vi "CSDB_Config.main.vi"(5 "error in (no error)":errorcluster) -> ()   [LabVIEW 2014, in "CSDB_Config.lvlib"]
doc: "Main User Panel"
uses:
  CSDB_Config.lvlib
panel:
  in  "select all":bool
  in  "delete instances":bool
  in  "cFilter :":string caption="Filter :"
  in  "createCSVFile4SVs":bool
  in  "Filter :":string
  out "Selected Instance :":string
  in  "edit selected instances":bool
  out "error out":errorcluster
  in  "exit":bool
  in  "createWithDefault":bool
  in  "create":bool
  in  "Preview":i32(listbox)
  in  "Instances":i32[](listbox)
  in  "Classes":i32(listbox)
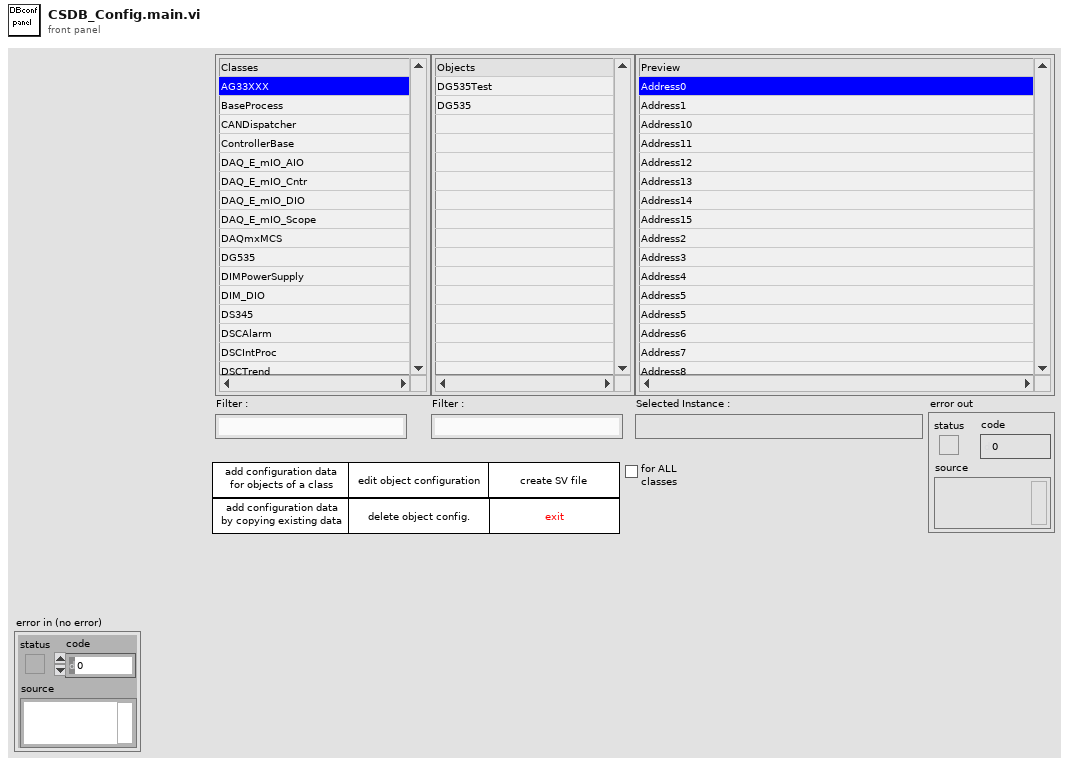
[diagram p1: front panel]
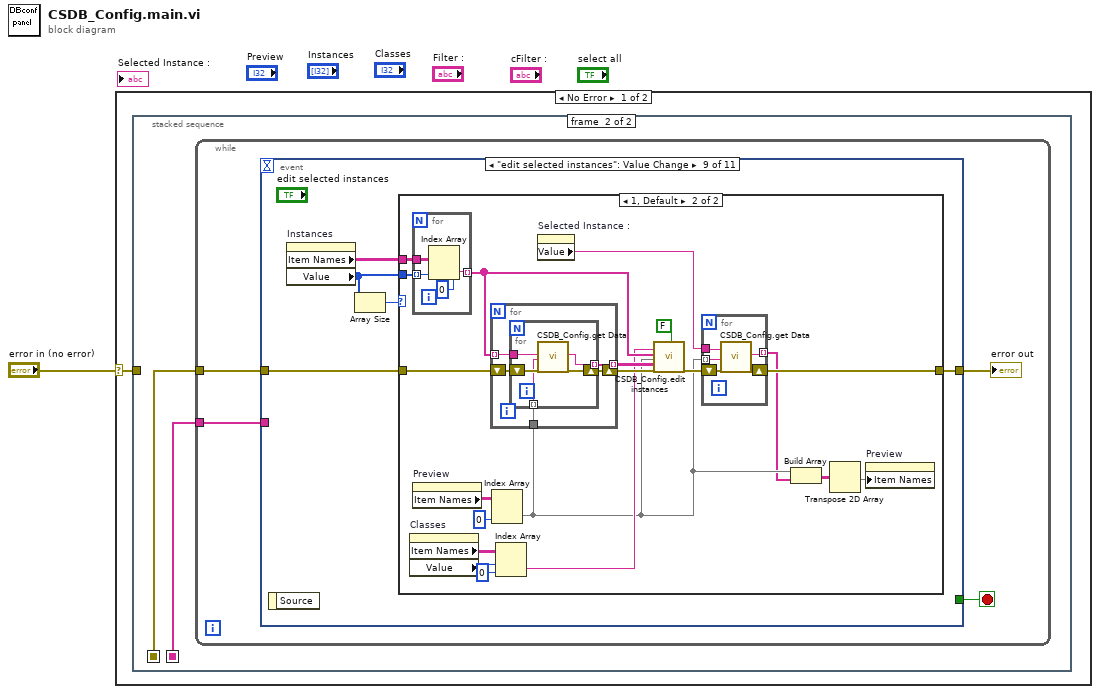
[diagram p0: block diagram]
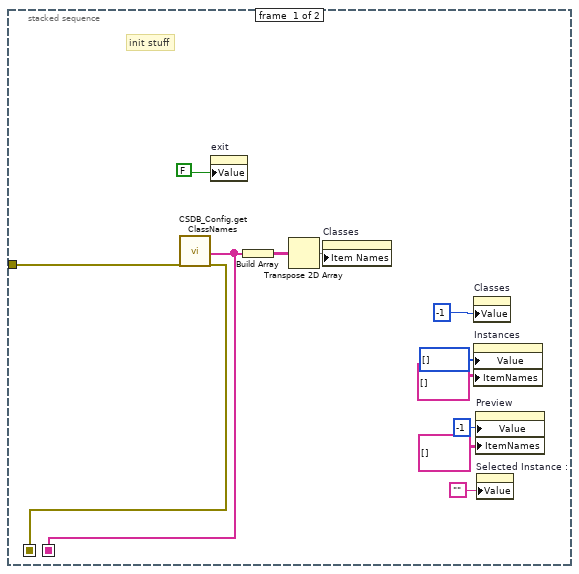
[diagram p2: hidden frame]
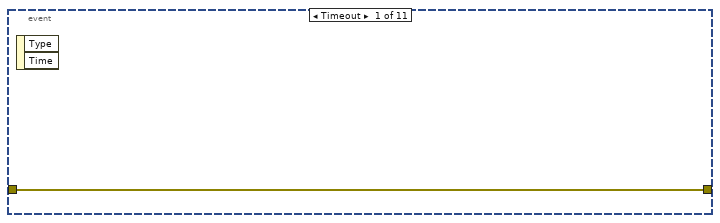
[diagram p3: hidden frame]
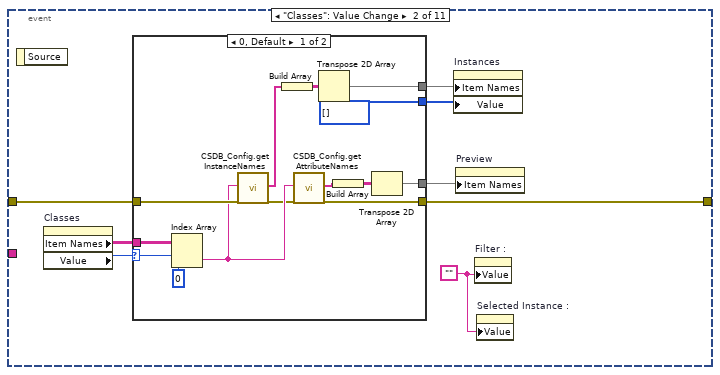
[diagram p4: hidden frame]
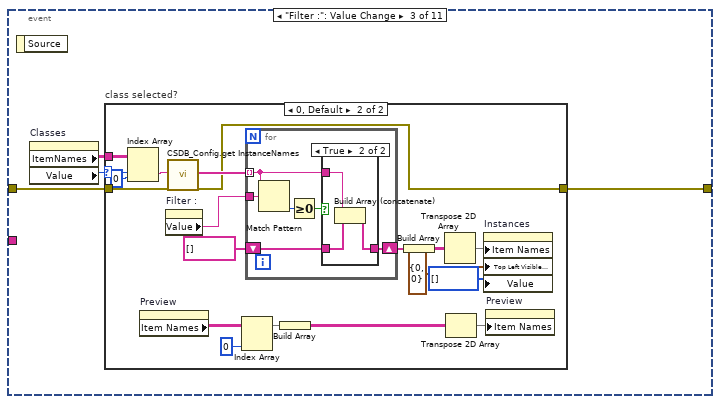
[diagram p6: hidden frame]
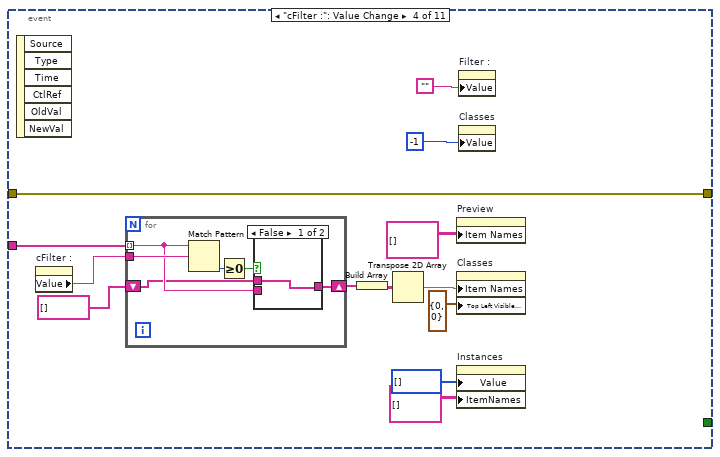
[diagram p9: hidden frame]
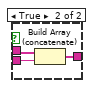
[diagram p10: hidden frame]
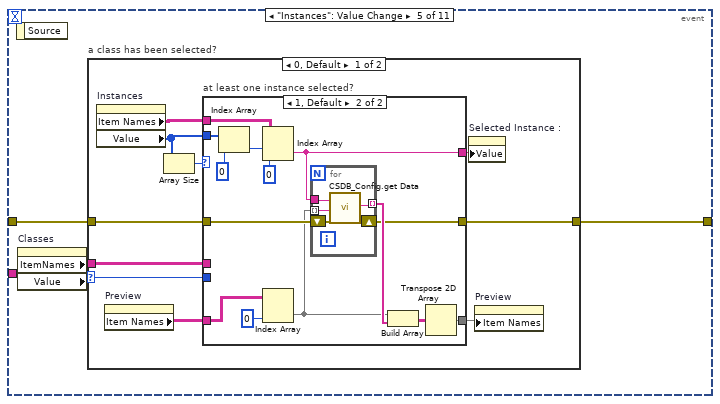
[diagram p11: hidden frame]
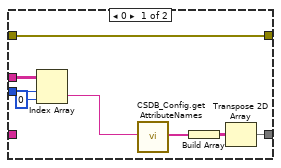
[diagram p12: hidden frame]
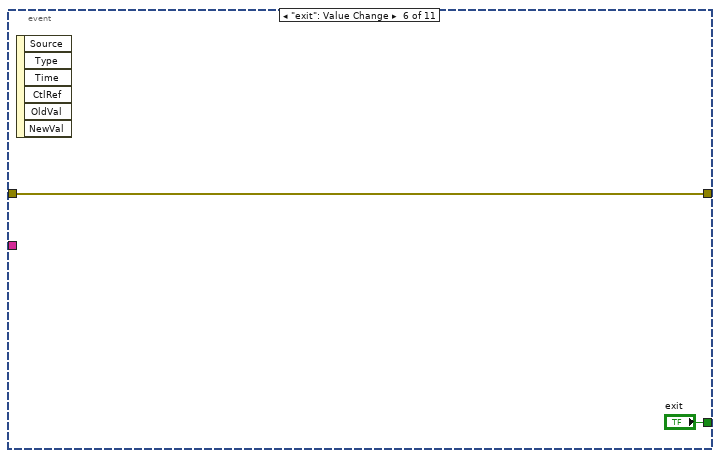
[diagram p14: hidden frame]
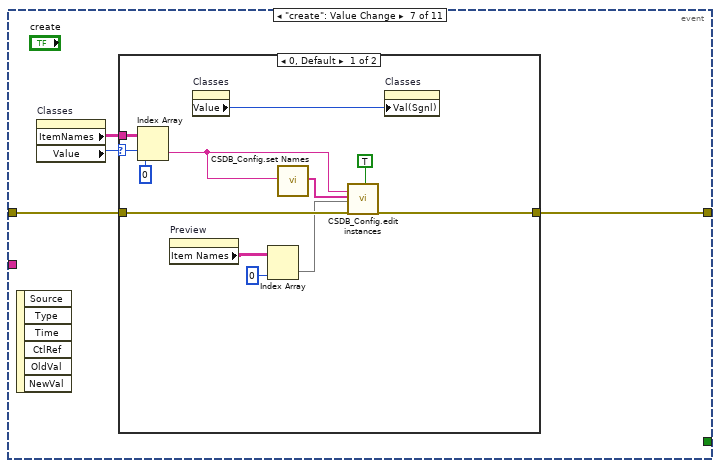
[diagram p15: hidden frame]
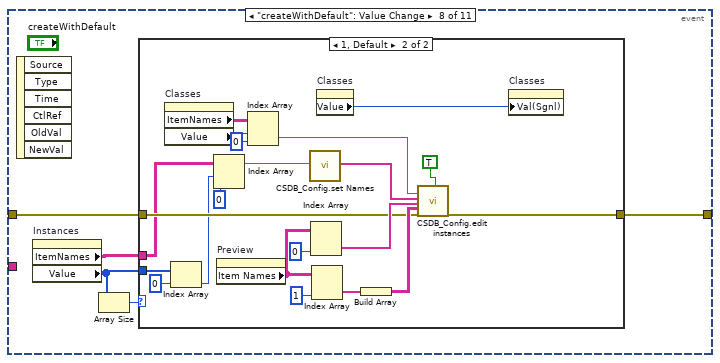
[diagram p17: hidden frame]
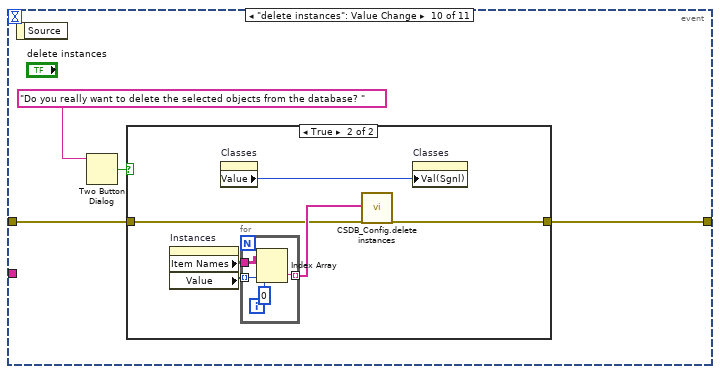
[diagram p20: hidden frame]
diagram:
  n1 = case shown="No Error" "error in (no error)" {
    selector: "error in (no error)" -> [w2 w288]
    frame No Error {
      n2 = stacked-sequence {
        seq-local: [w12 _] -> [_ w16]
        seq-local: [w7 _] -> [_ w15]
        tunnel: w2 -> [w13 _]
        frame #0 {
          # "init stuff"
          n3 = call "CSDB_Config.get ClassNames.vi"("error in (no error)"=w13) -> ("ClassNames"=w7:string[], "error out"=w12:errorcluster)  [unwired: 17 in]
          n4 = property on="exit" class="Bool"("Value"=FALSE) -> ()  [unwired: 2 in, 2 out]
          n5 = Build Array(w7) -> (w6:string[][])
          n6 = Transpose 2D Array(2D array=w6) -> (transposed array=w14:string[][])
          n7 = property on="Classes" class="MCListbox (strict)"("Item Names"=w14) -> ()  [unwired: 2 in, 2 out]
          n8 = property on="Classes" class="MCListbox (strict)"("Value"=-1 ("Classes")) -> ()  [unwired: 2 in, 2 out]
          n9 = property on="Instances" class="MCListbox (strict)"("Value"=i32[] [] ("Instances"), "ItemNames"=string[][] [] ("Item Names")) -> ()  [unwired: 2 in, 2 out]
          n10 = property on="Preview" class="MCListbox (strict)"("Value"=-1 ("Preview"), "ItemNames"=string[][] [] ("Item Names")) -> ()  [unwired: 2 in, 2 out]
          n11 = property on="Selected Instance :" class="Str"("Value"="") -> ()  [unwired: 2 in, 2 out]
        }
        frame #1 {
          n12 = while {
            tunnel: w16 -> [w19]
            tunnel: w15 -> [w18]
            stop <- w20 stop-if-true
            n13 = event shown="[8] \"edit selected instances\": Value Change" {
              selector: _ -> [_ _ _ _ _ _ _ _ _ _ _]
              dyn-events: _ -> [_ _ _ _ _ _ _ _ _ _ _]
              timeout: _ -> [_ _ _ _ _ _ _ _ _ _ _]
              tunnel: [_ _ _ _ _ "exit" _ _ _ _ _] -> w20
              tunnel: w19 -> [w21 w28 w48 w79 w105 w144 w149 w167 w193 w238 w253]
              tunnel: w18 -> [_ _ _ w91 _ _ _ _ _ _ w255]
              tunnel: [w21 w27 w45 w79 w103 w144 w146 w163 w190 w235 w251] -> w17
              event Timeout {
                n14 = event-data() -> ()  [unwired: 1 in, 2 out]
              }
              event "Classes": Value Change {
                w23 = ""
                n15 = event-data() -> ()  [unwired: 1 in, 1 out]
                n16 = property on="Classes" class="MCListbox (strict)"() -> ("Item Names"=w29:string[][], "Value"=w22:i32)  [unwired: 2 in, 2 out]
                n17 = case shown="0, Default" w22 {
                  selector: w22 -> [w30 _]
                  tunnel: w29 -> [w43 _]
                  tunnel: w28 -> [w42 w44]
                  tunnel: [w41 w44] -> w27
                  tunnel: [w37 _] -> w26
                  tunnel: [i32[] [] ("Instances") _] -> w25
                  tunnel: [w32 _] -> w24
                  frame 0, Default {
                    n18 = Index Array(array=w43, index (row)=w30, index (col)=0 ("disabled index (col)")) -> (element=w35:string)
                    n19 = call "CSDB_Config.get InstanceNames.vi"("ClassName"=w35, "error in (no error)"=w42) -> ("InstanceNames"=w39:string[], "error out"=w31:errorcluster)  [unwired: 16 in]
                    n20 = Build Array(w39) -> (w38:string[][])
                    n21 = call "CSDB_Config.get AttributeNames.vi"("ClassName"=w35, "error in (no error)"=w31) -> ("Attribute"=w34:string[], "error out"=w41:errorcluster)  [unwired: 16 in]
                    n22 = Transpose 2D Array(2D array=w38) -> (transposed array=w37:string[][])
                    n23 = Build Array(w34) -> (w33:string[][])
                    n24 = Transpose 2D Array(2D array=w33) -> (transposed array=w32:string[][])
                  }
                  frame -1 {
                  }
                }
                n25 = property on="Instances" class="MCListbox (strict)"("Item Names"=w26, "Value"=w25) -> ()  [unwired: 2 in, 2 out]
                n26 = property on="Preview" class="MCListbox (strict)"("Item Names"=w24) -> ()  [unwired: 2 in, 2 out]
                n27 = property on="Filter :" class="Str"("Value"=w23) -> ()  [unwired: 2 in, 2 out]
                n28 = property on="Selected Instance :" class="Str"("Value"=w23) -> ()  [unwired: 2 in, 2 out]
              }
              event "Filter :": Value Change {
                n29 = event-data() -> ()  [unwired: 1 in, 1 out]
                n30 = property on="Classes" class="MCListbox (strict)"() -> ("ItemNames"=w46:string[][], "Value"=w47:i32)  [unwired: 2 in, 2 out]
                n31 = case "class selected?" shown="0, Default" w47 {
                  selector: w47 -> [_ w59]
                  tunnel: w48 -> [w49 w68]
                  tunnel: w46 -> [_ w60]
                  tunnel: [w49 w50] -> w45
                  frame -1 {
                  }
                  frame 0, Default {
                    n32 = Index Array(array=w60, index (row)=w59, index (col)=0 ("disabled index (col)")) -> (element=w57:string)
                    n33 = property on="Preview" class="MCListbox (strict)"() -> ("Item Names"=w55:string[][])  [unwired: 2 in, 2 out]
                    n34 = property on="Filter :" class="Str"() -> ("Value"=w56:string)  [unwired: 2 in, 2 out]
                    n35 = call "CSDB_Config.get InstanceNames.vi"("ClassName"=w57, "error in (no error)"=w68) -> ("InstanceNames"=w67:string[], "error out"=w50:errorcluster)  [unwired: 16 in]
                    n36 = Index Array(array=w55, index (col)=0 ("disabled index (col)")) -> (element=w53:string[])  [unwired: 1 in]
                    n37 = for {
                      tunnel: w67 -> [w71] mode=indexing
                      tunnel: w56 -> [w74]
                      shift-right: [w69] -> w64
                      shift-left: string[] [] -> [w70]
                      n38 = Match Pattern(string=w71, regular expression=w74) -> (offset past match=w73:i32)  [unwired: 1 in, 3 out]
                      n39 = Greater Or Equal To 0?(x=w73) -> (x >= 0?=w72:bool)
                      n40 = case shown="True" w72 {
                        tunnel: w71 -> [_ w78]
                        tunnel: w70 -> [w75 w77]
                        tunnel: [w75 w76] -> w69
                        frame False {
                        }
                        frame True {
                          n41 = Build Array (concatenate)(w77, w78) -> (w76:string[])
                        }
                      }
                    }
                    n42 = Build Array(w53) -> (w52:string[][])
                    n43 = Build Array(w64) -> (w65:string[][])
                    n44 = Transpose 2D Array(2D array=w65) -> (transposed array=w63:string[][])
                    n45 = Transpose 2D Array(2D array=w52) -> (transposed array=w51:string[][])
                    n46 = property on="Instances" class="MCListbox (strict)"("Item Names"=w63, "Top Left Visible Cell"=cluster{"Row":u32, "Column":u32} {"Row"=0, "Column"=0}, "Value"=i32[] [] ("Instances")) -> ()  [unwired: 2 in, 2 out]
                    n47 = property on="Preview" class="MCListbox (strict)"("Item Names"=w51) -> ()  [unwired: 2 in, 2 out]
                  }
                }
              }
              event "cFilter :": Value Change {
                n48 = event-data() -> ()  [unwired: 1 in, 6 out]
                n49 = property on="cFilter :" class="Str"() -> ("Value"=w80:string)  [unwired: 2 in, 2 out]
                n50 = for {
                  tunnel: w91 -> [w94] mode=indexing
                  tunnel: w80 -> [w97]
                  shift-right: [w93] -> w88
                  shift-left: string[] [] -> [w92]
                  n51 = Match Pattern(string=w94, regular expression=w97) -> (offset past match=w96:i32)  [unwired: 1 in, 3 out]
                  n52 = Greater Or Equal To 0?(x=w96) -> (x >= 0?=w95:bool)
                  n53 = case shown="False" w95 {
                    tunnel: w94 -> [_ w101]
                    tunnel: [w98 w100] -> w93
                    tunnel: w92 -> [w98 w99]
                    frame False {
                    }
                    frame True {
                      n54 = Build Array (concatenate)(w99, w101) -> (w100:string[])
                    }
                  }
                }
                n55 = Build Array(w88) -> (w89:string[][])
                n56 = Transpose 2D Array(2D array=w89) -> (transposed array=w87:string[][])
                n57 = property on="Preview" class="MCListbox (strict)"("Item Names"=string[][] []) -> ()  [unwired: 2 in, 2 out]
                n58 = property on="Classes" class="MCListbox (strict)"("Item Names"=w87, "Top Left Visible Cell"=cluster{"Row":u32, "Column":u32} {"Row"=0, "Column"=0}) -> ()  [unwired: 2 in, 2 out]
                n59 = property on="Instances" class="MCListbox (strict)"("Value"=i32[] [] ("Instances"), "ItemNames"=string[][] [] ("Item Names")) -> ()  [unwired: 2 in, 2 out]
                n60 = property on="Filter :" class="Str"("Value"="") -> ()  [unwired: 2 in, 2 out]
                n61 = property on="Classes" class="MCListbox (strict)"("Value"=-1 ("Classes")) -> ()  [unwired: 2 in, 2 out]
              }
              event "Instances": Value Change {
                n62 = event-data() -> ()  [unwired: 1 in, 1 out]
                n63 = property on="Classes" class="MCListbox (strict)"() -> ("ItemNames"=w102:string[][], "Value"=w104:i32)  [unwired: 2 in, 2 out]
                n64 = case "a class has been selected?" shown="0, Default" w104 {
                  selector: w104 -> [w106 _]
                  tunnel: w105 -> [w114 w143]
                  tunnel: [w111 w143] -> w103
                  tunnel: w102 -> [w107 _]
                  frame 0, Default {
                    n65 = property on="Instances" class="MCListbox (strict)"() -> ("Item Names"=w115:string[][], "Value"=w109:i32[])  [unwired: 2 in, 2 out]
                    n66 = property on="Preview" class="MCListbox (strict)"() -> ("Item Names"=w108:string[][])  [unwired: 2 in, 2 out]
                    n67 = Array Size(array=w109) -> (size(s)=w110:i32)
                    n68 = case "at least one instance selected?" shown="1, Default" w110 {
                      tunnel: w115 -> [_ w137]
                      tunnel: w114 -> [w123 w135]
                      tunnel: [w120 w132] -> w113
                      tunnel: [_ w129] -> w112
                      tunnel: w109 -> [_ w128]
                      tunnel: [w123 w125] -> w111
                      tunnel: w108 -> [_ w124]
                      tunnel: w107 -> [w119 _]
                      tunnel: w106 -> [w118 _]
                      frame 0 {
                        n69 = Index Array(array=w119, index (row)=w118, index (col)=0 ("disabled index (col)")) -> (element=w116:string)
                        n70 = call "CSDB_Config.get AttributeNames.vi"("ClassName"=w116) -> ("Attribute"=w122:string[])  [unwired: 17 in, 1 out]
                        n71 = Build Array(w122) -> (w121:string[][])
                        n72 = Transpose 2D Array(2D array=w121) -> (transposed array=w120:string[][])
                      }
                      frame 1, Default {
                        n73 = Index Array(array=w128, index=0) -> (element=w131:i32)
                        n74 = Index Array(array=w137, index (row)=w131, index (col)=0 ("disabled index (col)")) -> (element=w129:string)
                        n75 = Index Array(array=w124, index (col)=0 ("disabled index (col)")) -> (element=w126:string[])  [unwired: 1 in]
                        n76 = for {
                          tunnel: w129 -> [w141]
                          tunnel: w126 -> [w140] mode=indexing
                          tunnel: [w139] -> w134 mode=indexing
                          shift-right: [w138] -> w125
                          shift-left: w135 -> [w142]
                          n77 = call "CSDB_Config.get Data.vi"("InstanceName"=w141, "AttributeName"=w140, "error in (no error)"=w142) -> ("Value"=w139:string, "error out"=w138:errorcluster)  [unwired: 15 in]
                        }
                        n78 = Build Array(w126, w134) -> (w133:string[][])
                        n79 = Transpose 2D Array(2D array=w133) -> (transposed array=w132:string[][])
                      }
                    }
                    n80 = property on="Selected Instance :" class="Str"("Value"=w112) -> ()  [unwired: 2 in, 2 out]
                    n81 = property on="Preview" class="MCListbox (strict)"("Item Names"=w113) -> ()  [unwired: 2 in, 2 out]
                  }
                  frame -1 {
                  }
                }
              }
              event "exit": Value Change {
                n82 = event-data() -> ()  [unwired: 1 in, 6 out]
              }
              event "create": Value Change {
                n83 = event-data() -> ()  [unwired: 1 in, 6 out]
                n84 = property on="Classes" class="MCListbox (strict)"() -> ("ItemNames"=w147:string[][], "Value"=w148:i32)  [unwired: 2 in, 2 out]
                n85 = case shown="0, Default" w148 {
                  selector: w148 -> [w157 _]
                  tunnel: w149 -> [w159 w162]
                  tunnel: w147 -> [w158 _]
                  tunnel: [w151 w162] -> w146
                  frame 0, Default {
                    n86 = Index Array(array=w158, index (row)=w157, index (col)=0 ("disabled index (col)")) -> (element=w155:string)
                    n87 = property on="Preview" class="MCListbox (strict)"() -> ("Item Names"=w154:string[][])  [unwired: 2 in, 2 out]
                    n88 = property on="Classes" class="MCListbox (strict)"() -> ("Value"=w150:i32)  [unwired: 2 in, 2 out]
                    n89 = Index Array(array=w154, index (col)=0 ("disabled index (col)")) -> (element=w152:string[])  [unwired: 1 in]
                    n90 = call "CSDB_Config.set Names.vi"("Name"=w155) -> ("Names"=w161:string[])  [unwired: 18 in]
                    n91 = call "CSDB_Config.edit instances.vi"("Classname"=w155, "Names"=w161, "Attributes"=w152, "error in (no error)"=w159, "new instances?"=TRUE) -> ("error out"=w151:errorcluster)  [unwired: 14 in]
                    n92 = property on="Classes" class="MCListbox (strict)"("Val(Sgnl)"=w150) -> ()  [unwired: 2 in, 2 out]
                  }
                  frame -1 {
                  }
                }
              }
              event "createWithDefault": Value Change {
                n93 = event-data() -> ()  [unwired: 1 in, 6 out]
                n94 = property on="Instances" class="MCListbox (strict)"() -> ("ItemNames"=w164:string[][], "Value"=w165:i32[])  [unwired: 2 in, 2 out]
                n95 = Array Size(array=w165) -> (size(s)=w166:i32)
                n96 = case shown="1, Default" w166 {
                  tunnel: w167 -> [w168 w181]
                  tunnel: w165 -> [_ w178]
                  tunnel: w164 -> [_ w177]
                  tunnel: [w168 w170] -> w163
                  frame 0 {
                  }
                  frame 1, Default {
                    n97 = property on="Classes" class="MCListbox (strict)"() -> ("ItemNames"=w174:string[][], "Value"=w173:i32)  [unwired: 2 in, 2 out]
                    n98 = Index Array(array=w178, index=0) -> (element=w179:i32)
                    n99 = Index Array(array=w177, index (row)=w179, index (col)=0 ("disabled index (col)")) -> (element=w176:string)
                    n100 = property on="Preview" class="MCListbox (strict)"() -> ("Item Names"=w185:string[][])  [unwired: 2 in, 2 out]
                    n101 = Index Array(array=w174, index (row)=w173, index (col)=0 ("disabled index (col)")) -> (element=w171:string)
                    n102 = call "CSDB_Config.set Names.vi"("Name"=w176) -> ("Names"=w189:string[])  [unwired: 18 in]
                    n103 = Index Array(array=w185, index (col)=0 ("disabled index (col)")) -> (element=w188:string[])  [unwired: 1 in]
                    n104 = Index Array(array=w185, index (col)=1 ("disabled index (col)")) -> (element=w184:string[])  [unwired: 1 in]
                    n105 = property on="Classes" class="MCListbox (strict)"() -> ("Value"=w169:i32)  [unwired: 2 in, 2 out]
                    n106 = Build Array(w184) -> (w183:string[][])
                    n107 = call "CSDB_Config.edit instances.vi"("Classname"=w171, "Names"=w189, "Attributes"=w188, "Values"=w183, "error in (no error)"=w181, "new instances?"=TRUE) -> ("error out"=w170:errorcluster)  [unwired: 13 in]
                    n108 = property on="Classes" class="MCListbox (strict)"("Val(Sgnl)"=w169) -> ()  [unwired: 2 in, 2 out]
                  }
                }
              }
              event "edit selected instances": Value Change {
                n109 = event-data() -> ()  [unwired: 1 in, 1 out]
                n110 = property on="Instances" class="MCListbox (strict)"() -> ("Item Names"=w194:string[][], "Value"=w192:i32[])  [unwired: 2 in, 2 out]
                n111 = Array Size(array=w192) -> (size(s)=w191:i32)
                n112 = case shown="1, Default" w191 {
                  tunnel: w192 -> [_ w215]
                  tunnel: w194 -> [_ w214]
                  tunnel: w193 -> [w195 w207]
                  tunnel: [w195 w201] -> w190
                  frame 0 {
                  }
                  frame 1, Default {
                    n113 = property on="Classes" class="MCListbox (strict)"() -> ("Item Names"=w206:string[][], "Value"=w205:i32)  [unwired: 2 in, 2 out]
                    n114 = for {
                      tunnel: w215 -> [w233] mode=indexing
                      tunnel: w214 -> [w234]
                      tunnel: [w231] -> w210 mode=indexing
                      n115 = Index Array(array=w234, index (row)=w233, index (col)=0 ("disabled index (col)")) -> (element=w231:string)
                    }
                    n116 = property on="Preview" class="MCListbox (strict)"() -> ("Item Names"=w213:string[][])  [unwired: 2 in, 2 out]
                    n117 = Index Array(array=w213, index (col)=0 ("disabled index (col)")) -> (element=w198:string[])  [unwired: 1 in]
                    n118 = for {
                      tunnel: w210 -> [w223] mode=indexing
                      tunnel: w198 -> [w222]
                      tunnel: [w221] -> w209 mode=indexing
                      shift-right: [w224] -> w211
                      shift-left: w207 -> [w225]
                      n119 = for {
                        tunnel: w223 -> [w228]
                        tunnel: w222 -> [w227] mode=indexing
                        tunnel: [w226] -> w221 mode=indexing
                        shift-right: [w229] -> w224
                        shift-left: w225 -> [w230]
                        n120 = call "CSDB_Config.get Data.vi"("InstanceName"=w228, "AttributeName"=w227, "error in (no error)"=w230) -> ("Value"=w226:string, "error out"=w229:errorcluster)  [unwired: 15 in]
                      }
                    }
                    n121 = Index Array(array=w206, index (row)=w205, index (col)=0 ("disabled index (col)")) -> (element=w203:string)
                    n122 = property on="Selected Instance :" class="Str"() -> ("Value"=w200:string)  [unwired: 2 in, 2 out]
                    n123 = call "CSDB_Config.edit instances.vi"("Classname"=w203, "Names"=w210, "Attributes"=w198, "Values"=w209, "error in (no error)"=w211, "new instances?"=FALSE) -> ("error out"=w202:errorcluster)  [unwired: 13 in]
                    n124 = for {
                      tunnel: w200 -> [w219]
                      tunnel: w198 -> [w218] mode=indexing
                      tunnel: [w217] -> w197 mode=indexing
                      shift-right: [w216] -> w201
                      shift-left: w202 -> [w220]
                      n125 = call "CSDB_Config.get Data.vi"("InstanceName"=w219, "AttributeName"=w218, "error in (no error)"=w220) -> ("Value"=w217:string, "error out"=w216:errorcluster)  [unwired: 15 in]
                    }
                    n126 = Build Array(w198, w197) -> (w199:string[][])
                    n127 = Transpose 2D Array(2D array=w199) -> (transposed array=w196:string[][])
                    n128 = property on="Preview" class="MCListbox (strict)"("Item Names"=w196) -> ()  [unwired: 2 in, 2 out]
                  }
                }
              }
              event "delete instances": Value Change {
                n129 = event-data() -> ()  [unwired: 1 in, 1 out]
                n130 = Two Button Dialog(message="Do you really want to delete the selected objects from the database? ") -> (T button?=w237:bool)  [unwired: 2 in]
                n131 = case shown="True" w237 {
                  tunnel: w238 -> [w239 w242]
                  tunnel: [w239 w241] -> w235
                  frame False {
                  }
                  frame True {
                    n132 = property on="Instances" class="MCListbox (strict)"() -> ("Item Names"=w244:string[][], "Value"=w245:i32[])  [unwired: 2 in, 2 out]
                    n133 = property on="Classes" class="MCListbox (strict)"() -> ("Value"=w240:i32)  [unwired: 2 in, 2 out]
                    n134 = for {
                      tunnel: w245 -> [w248] mode=indexing
                      tunnel: w244 -> [w249]
                      tunnel: [w246] -> w243 mode=indexing
                      n135 = Index Array(array=w249, index (row)=w248, index (col)=0 ("disabled index (col)")) -> (element=w246:string)
                    }
                    n136 = call "CSDB_Config.delete instances.vi"("Names"=w243, "error in (no error)"=w242) -> ("error out"=w241:errorcluster)  [unwired: 17 in]
                    n137 = property on="Classes" class="MCListbox (strict)"("Val(Sgnl)"=w240) -> ()  [unwired: 2 in, 2 out]
                  }
                }
              }
              event "createCSVFile4SVs": Value Change {
                n138 = event-data() -> ()  [unwired: 1 in, 6 out]
                n139 = property on="select all" class="Bool (strict)"() -> ("Value"=w250:bool)  [unwired: 2 in, 2 out]
                n140 = case "for ALL objects?" shown="False" w250 {
                  tunnel: [w262 w276] -> w256
                  tunnel: w255 -> [_ w277]
                  tunnel: cluster{string, string}[] [] -> [_ w275]
                  tunnel: w253 -> [w257 w274]
                  tunnel: [w257 w273] -> w252
                  frame False {
                    n141 = property on="Instances" class="MCListbox (strict)"() -> ("Item Names"=w265:string[][], "Value"=w264:i32[])  [unwired: 2 in, 2 out]
                    n142 = property on="Classes" class="MCListbox (strict)"() -> ("ItemNames"=w261:string[][], "Value"=w260:i32)  [unwired: 2 in, 2 out]
                    n143 = for {
                      tunnel: w264 -> [w271] mode=indexing
                      tunnel: w265 -> [w272]
                      tunnel: [w269] -> w263 mode=indexing
                      n144 = Index Array(array=w272, index (row)=w271, index (col)=0 ("disabled index (col)")) -> (element=w269:string)
                    }
                    n145 = Index Array(array=w261, index (row)=w260, index (col)=0 ("disabled index (col)")) -> (element=w258:string)
                    n146 = for {
                      tunnel: w263 -> [w268] mode=indexing
                      tunnel: w258 -> [w266]
                      tunnel: [w267] -> w262 mode=indexing
                      n147 = Bundle(w268, w266) -> (w267:cluster{string, string})  [unwired: 1 in]
                    }
                  }
                  frame True {
                    n148 = for {
                      tunnel: w277 -> [w283] mode=indexing
                      shift-right: [w281] -> w276
                      shift-left: w275 -> [w280]
                      shift-right: [w278] -> w273
                      shift-left: w274 -> [w279]
                      n149 = call "CSDB_Config.get InstanceNames.vi"("ClassName"=w283, "error in (no error)"=w279) -> ("InstanceNames"=w284:string[], "error out"=w278:errorcluster)  [unwired: 16 in]
                      n150 = for {
                        tunnel: w284 -> [w287] mode=indexing
                        tunnel: w283 -> [w285]
                        tunnel: [w286] -> w282 mode=indexing
                        n151 = Bundle(w287, w285) -> (w286:cluster{string, string})  [unwired: 1 in]
                      }
                      n152 = Build Array (concatenate)(w280, w282) -> (w281:cluster{string, string}[])
                    }
                  }
                }
                n153 = call "CSDB_Config.write SV CSV-file.vi"("objects"=w256, "error in"=w252) -> ("error out"=w251:errorcluster)  [unwired: 17 in]
              }
            }
            "error out" <- w17
          }
        }
      }
    }
    frame Error {
      n154 = property on="error out" class="Clust (strict)"("Value"=w288) -> ()  [unwired: 2 in, 2 out]
    }
  }
